vi "SubFuzzy2.vi"(8 "error in (no error)":errorcluster, 11 "input values":dbl[](array[numeric])) -> (0 "error out":errorcluster, 3 "output values":dbl[](array[numeric]))   [LabVIEW 2014]
uses:
  <vilib>/addons/Fuzzy Logic/FL Fuzzy Controller (MIMO).vi
  <vilib>/addons/Fuzzy Logic/NI_Fuzzy_Logic_API.lvlib
panel:
  in  "Stop":bool
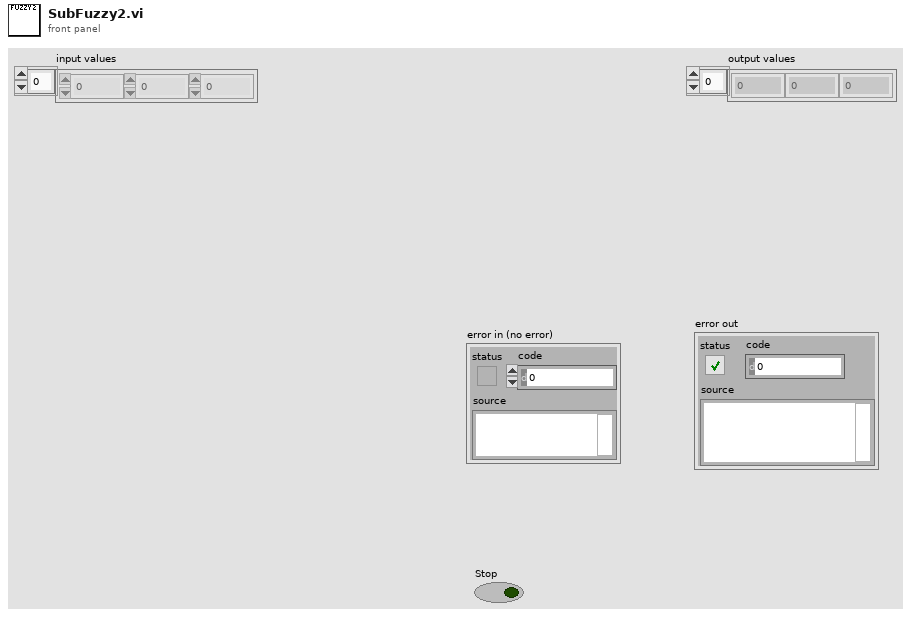
[diagram p1: front panel]
types:
  T1 = typedef "NI_Fuzzy_Logic_API.lvlib/FL System.ctl" = cluster{"input variables":T2[], "output variables":T2[], "rules":T5[], "defuzzification method":T11, "description":string, "user MF interpolating polynomials":T12[]}
  T2 = typedef "NI_Fuzzy_Logic_API.lvlib/FL Variable.ctl" = cluster{"name":string, "range":dbl[], "MFs":T3[]}
  T3 = typedef "NI_Fuzzy_Logic_API.lvlib/FL Membership Function.ctl" = cluster{"name":string, "shape":T4, "points":dbl[], "color":u32, "user-defined shape index":i32}
  T4 = typedef "NI_Fuzzy_Logic_API.lvlib/FL Membership Function Shape.ctl" = u16
  T5 = typedef "NI_Fuzzy_Logic_API.lvlib/FL Rule.ctl" = cluster{"antecedents":T6[], "antecedent connective":T8, "consequents":T9[], "consequent implication":T10, "degree of support":dbl}
  T6 = typedef "NI_Fuzzy_Logic_API.lvlib/FL Antecedent.ctl" = cluster{"Var Index":i32, "MF Index":i32, "Cond":T7}
  T7 = typedef "NI_Fuzzy_Logic_API.lvlib/FL Modifier.ctl" = u16
  T8 = typedef "NI_Fuzzy_Logic_API.lvlib/FL Antecedent Connective.ctl" = u16
  T9 = typedef "NI_Fuzzy_Logic_API.lvlib/FL Consequent.ctl" = cluster{"Var Index":i32, "MF Index":i32, "Cond":T7}
  T10 = typedef "NI_Fuzzy_Logic_API.lvlib/FL Consequent Implication.ctl" = u16
  T11 = typedef "NI_Fuzzy_Logic_API.lvlib/FL Defuzzification.ctl" = u16
  T12 = typedef "NI_Fuzzy_Logic_API.lvlib/FL Interpolating polynomials.ctl" = cluster{"X":dbl[], "Y":dbl[], "Y(x) coeff":dbl[][], "X(y) coeff":dbl[][], "Area(y) coeff":dbl[][], "coa_x(y) coeff":dbl[][]}
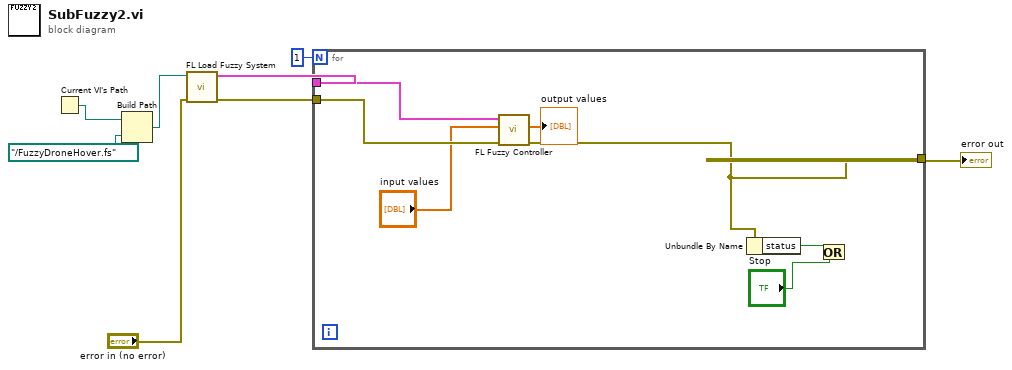
[diagram p0: block diagram]
diagram:
  n1 = Current VI's Path() -> (path=w8:path)
  n2 = Build Path(base path=w8, name or relative path=path "../FuzzyDroneHover.fs") -> (appended path=w6:path)
  n3 = call <vilib>:"FL Load Fuzzy System.vi"("error in (no error)"="error in (no error)", "file path"=w6) -> ("error out"=w4:errorcluster, "fuzzy system out"=w5:T1)  [unwired: 8 in]
  n4 = for {
    N: 1 -> [_]
    tunnel: w5 -> [w15]
    tunnel: w4 -> [w14]
    tunnel: [w11] -> w3
    n5 = call-poly <vilib>:"FL Fuzzy Controller.vi"("error in (no error)"=w14, "input values"="input values", "fuzzy system in"=w15) -> ("error out"=w11:errorcluster, "output values"=→"output values":dbl[])  [unwired: 4 in, 3 out]
    n6 = Unbundle By Name(w11) -> ("status"=w13:bool)
    n7 = Or(x=w13, y="Stop") -> ()  [unwired: 1 out]
  }
  "error out" <- w3
